vi "Main.vi"() -> ()   [LabVIEW 2017]
doc: "The myRIO Project template acquires acceleration data from the onboard accelerometer and displays the changes of acceleration values in a waveform chart."
uses:
  <vilib>/myRIO/Common/Instrument Driver Framework/myRIO v1.0/IRQ/typedefs/DI IRQ Type.ctl
  <vilib>/Platform/TimedLoop/XDataNode/timing_clust.ctl
  <vilib>/Platform/TimedLoop/XDataNode/nitl_modes.ctl
  <vilib>/Platform/TimedLoop/XDataNode/wakeup.ctl
  <vilib>/myRIO/Common/Instrument Driver Framework/myRIO v1.0/Encoder/typedefs/Encoder Signal Mode.ctl
  <vilib>/myRIO/Instrument Drivers/Onboard IO/Encoder/typedefs/Encoder Reference.ctl
  <vilib>/myRIO/Common/Instrument Driver Framework/Utilities/typedefs/myRIO Generic Hardware Reference.ctl
  <vilib>/myRIO/Common/Instrument Driver Framework/Utilities/typedefs/Hardware Version Enum.ctl
  <vilib>/myRIO/Common/Instrument Driver Framework/Utilities/typedefs/myRIO v1.0 Reference.ctl
  <vilib>/myRIO/Common/Instrument Driver Framework/Utilities/typedefs/Generic FPGA Reference.ctl
  <vilib>/myRIO/Common/Instrument Driver Framework/myRIO v1.0/Encoder/typedefs/Encoder Channels Enum.ctl
  <vilib>/myRIO/Common/Instrument Driver Framework/myRIO v1.0/Encoder/typedefs/Encoder Configuration v1.0.ctl
  <vilib>/userdefined/High Color/nirio_resource_hc.ctl
  <vilib>/myRIO/Instrument Drivers/Onboard IO/DIO/typedefs/DIO Reference.ctl
  <vilib>/myRIO/Common/Instrument Driver Framework/myRIO v1.0/DIO/typedefs/DIO Channels List.ctl
  <vilib>/myRIO/Common/Instrument Driver Framework/myRIO v1.0/DIO/typedefs/DIO Channels Enum.ctl
  <vilib>/myRIO/Instrument Drivers/Onboard Devices/Accelerometer/typedefs/Accelerometer Reference.ctl
  <vilib>/myRIO/Common/Instrument Driver Framework/myRIO v1.0/Accelerometer/typedefs/Accelerometer Channels List.ctl
  <vilib>/myRIO/Common/Instrument Driver Framework/myRIO v1.0/Accelerometer/typedefs/Accelerometer Channels Enum.ctl
  <vilib>/myRIO/Common/Instrument Driver Framework/Utilities/vis/Is FPGA Ref Available.vi
  <vilib>/myRIO/Common/Instrument Driver Framework/myRIO v1.0/Encoder/vis/myRIO v1.1 Open Encoder.vi
  <vilib>/myRIO/Instrument Drivers/Onboard IO/Encoder/vis/Read.vi
  <vilib>/myRIO/Common/Instrument Driver Framework/myRIO v1.0/Accelerometer/vis/myRIO v1.1 Open Accelerometer.vi
  <vilib>/myRIO/Instrument Drivers/Onboard Devices/Accelerometer/vis/Read.vi
  <vilib>/myRIO/Common/Instrument Driver Framework/myRIO v1.0/DIO/vis/myRIO v1.1 Open DIO.vi
  <vilib>/myRIO/Instrument Drivers/Onboard IO/DIO/vis/Read.vi
  <vilib>/myRIO/Instrument Drivers/Onboard IO/DIO/vis/Write.vi
  <vilib>/myRIO/Common/Instrument Driver Framework/Utilities/vis/Validate Channels.vi
  <vilib>/myRIO/Common/Instrument Driver Framework/myRIO v1.0/Encoder/vis/myRIO v1.0 Reserve Encoder.vi
  <vilib>/myRIO/Common/Instrument Driver Framework/myRIO v1.0/UART/vis/myRIO v1.0 Close UART.vi
  <vilib>/myRIO/Common/Instrument Driver Framework/myRIO v1.0/Accelerometer/vis/myRIO v1.0 Reserve Accelerometer.vi
  <vilib>/myRIO/Common/Instrument Driver Framework/myRIO v1.0/DIO/vis/myRIO v1.0 Reserve DIO.vi
  <vilib>/myRIO/Common/Instrument Driver Framework/myRIO v1.0/Encoder/vis/myRIO v1.0 Build MUX Configuration Encoder.vi
  <vilib>/myRIO/Common/Instrument Driver Framework/myRIO v1.0/Resource Manager/vis/myRIO v1.0 Reserve Channel List.vi
  <vilib>/myRIO/Common/Instrument Driver Framework/myRIO v1.0/Accelerometer/vis/myRIO v1.0 Build MUX Configuration Accelerometer.vi
  <vilib>/myRIO/Common/Instrument Driver Framework/myRIO v1.0/DIO/vis/myRIO v1.0 Build MUX Configuration DIO.vi
  <vilib>/myRIO/Common/Instrument Driver Framework/myRIO v1.0/Resource Manager/vis/myRIO v1.0 Create Configuration List.vi
  <vilib>/myRIO/Common/Instrument Driver Framework/myRIO v1.0/Resource Manager/vis/myRIO v1.0 Reserve Channel.vi
  <vilib>/myRIO/Common/Instrument Driver Framework/myRIO v1.0/Resource Manager/vis/myRIO v1.0 Unreserve Channel.vi
  <vilib>/myRIO/Common/Instrument Driver Framework/myRIO v1.0/Resource Manager/vis/myRIO v1.0 Build Mutex Name.vi
  global.vi
  <vilib>/Utility/VariantDataType/GetNumericInfo.vi
  <vilib>/Utility/error.llb/Error Cluster From Error Code.vi
  <vilib>/myRIO/Common/Instrument Driver Framework/myRIO v1.0/myRIO v1.1 Open.vi
  <vilib>/myRIO/Common/Instrument Driver Framework/Utilities/vis/IO Manager.vi
  <vilib>/myRIO/Common/Instrument Driver Framework/Utilities/vis/Configuration Manager.vi
  <vilib>/myRIO/Common/Instrument Driver Framework/myRIO v1.0/Resource Manager/vis/myRIO v1.0 Configure IO.vi
  <vilib>/myRIO/Common/Instrument Driver Framework/myRIO v1.0/myRIO v1.0 Close.vi
  <vilib>/myRIO/Common/Instrument Driver Framework/myRIO v1.0/Encoder/vis/myRIO v1.0 Configure Encoder.vi
  <vilib>/myRIO/Common/Instrument Driver Framework/myRIO v1.0/Encoder/vis/myRIO v1.0 Read Encoder.vi
  State2016.vi
  <vilib>/addons/control/pid/pid.llb/PID (DBL).vi
  <vilib>/myRIO/Common/Instrument Driver Framework/Utilities/vis/FPGA Ref Manager.vi
  <vilib>/myRIO/Common/Instrument Driver Framework/myRIO v1.0/myRIO v1.0 Reset FPGA.vi
  <vilib>/myRIO/Common/Instrument Driver Framework/myRIO v1.0/IRQ/vis/myRIO v1.0 IRQ Info FGV.vi
  <vilib>/myRIO/Common/Instrument Driver Framework/myRIO v1.0/IRQ/vis/myRIO v1.0 Timer IRQ Info FGV.vi
  <vilib>/myRIO/Common/Instrument Driver Framework/myRIO v1.0/IRQ/vis/myRIO v1.0 ISR Agent.vi
  motion_command.vi
  <vilib>/myRIO/Common/Instrument Driver Framework/myRIO v1.0/DIO/vis/myRIO v1.0 Write DIO.vi
  <vilib>/myRIO/Common/Instrument Driver Framework/myRIO v1.0/DIO/vis/myRIO v1.0 Read DIO.vi
  <vilib>/myRIO/Common/Instrument Driver Framework/myRIO v1.0/Accelerometer/vis/myRIO v1.0 Get Scaling Constant Accelerometer.vi
  <vilib>/myRIO/Common/Instrument Driver Framework/myRIO v1.0/Accelerometer/vis/myRIO v1.0 Read Accelerometer.vi
  <vilib>/myRIO/Common/Instrument Driver Framework/myRIO v1.0/IRQ/vis/myRIO v1.1 Register DI IRQ.vi
  <vilib>/Platform/TimedLoop/XDataNode/XDataNode.xnode
  <vilib>/myRIO/Express VI/Onboard IO/Encoder/Encoder Express VI.xnode
  <vilib>/myRIO/Instrument Drivers/Onboard IO/Encoder/vis/myRIO Encoder Open.xnode
  <vilib>/myRIO/Common/Instrument Driver Framework/myRIO v1.0/Encoder/typedefs/Encoder Count Direction Enum.ctl
  <vilib>/myRIO/Express VI/Onboard Devices/LED/LED Express VI.xnode
  <vilib>/myRIO/Instrument Drivers/Onboard IO/DIO/vis/myRIO DIO Open.xnode
  <vilib>/myRIO/Express VI/Onboard IO/DI/DI Express VI.xnode
  <vilib>/myRIO/Express VI/Onboard Devices/Accelerometer/Accelerometer Express VI.xnode
  <vilib>/myRIO/Instrument Drivers/Onboard Devices/Accelerometer/vis/myRIO Accelerometer Open.xnode
  <vilib>/myRIO/Instrument Drivers/IRQ/IO IRQ/vis/myRIO Register DI IRQ.xnode
  <vilib>/myRIO/Common/Instrument Driver Framework/myRIO v1.0/IRQ/typedefs/Callback VI Ref.ctl
  <vilib>/myRIO/Instrument Drivers/Utilities/Utilities.lvlib
  <vilib>/Platform/TimedLoop/XDataNode/XDNodeRunTimeDep.lvlib
  <vilib>/myRIO/Instrument Drivers/Onboard IO/Encoder/Encoder.lvlib
  <vilib>/addons/control/pid/NI_PID_pid.lvlib
  <vilib>/myRIO/Instrument Drivers/Onboard IO/DIO/DIO.lvlib
  <vilib>/myRIO/Instrument Drivers/Onboard Devices/Accelerometer/Accelerometer.lvlib
panel:
  in  "T/S":bool
  in  "Speed":dbl(slide) scale=0.0..1.0
  in  "Torque":dbl(slide) scale=0.0..500.0
  out "Motion\nCommand":bool
  out "S/T Control":bool
  in  "Speed scale":dbl=1.0 format="%#_13g"
  in  "Stop":bool
  out "error out 2":errorcluster
  in  "PID gains 2":T1={"proportional gain (Kc)"=150.0, "integral time (Ti, min)"=0.0005, "derivative time (Td, min)"=1e-06} caption="PID 게인" {"derivative time (Td, min)" format="%.6f"; "integral time (Ti, min)" format="%.4f"; "proportional gain (Kc)" format="%.3f"}
  out "웨이브폼 차트 2":cluster{"Speed":dbl, dbl, dbl}(graph)={"Speed"=0.003129890453834161, -6.70631856770996, 0.00312989045383416}
  out "m/s 2":dbl(knob)=6.70631856770996 scale=0.0..2.0
  out "RPS 2":dbl(knob)=14.23125 scale=0.0..5.0
  out "km/h 2":dbl(knob)=24.14274684375586 scale=0.0..10.0
  out "RPM 2":dbl(knob)=853.875 scale=0.25..250.0
  out "output 2":dbl=500.0
  out "CW 2":bool
  in  "ip 2":i32=77
  out "RC Control":bool
  out "CW":bool
  out "output":dbl=-44.009136764238946
  out "RPM":dbl(knob)=0.75 scale=0.25..250.0
  out "km/h":dbl(knob)=0.021205750411731103 scale=0.0..10.0
  out "RPS":dbl(knob)=0.0125 scale=0.0..5.0
  out "m/s":dbl(knob)=0.005890486225480862 scale=0.0..2.0
  out "웨이브폼 차트":cluster{"Speed":dbl, dbl, dbl}(graph)={"Speed"=0.003129890453834161, 0.005890486225480862, 0.00312989045383416}
  in  "PID gains":T1={"proportional gain (Kc)"=150.0, "integral time (Ti, min)"=0.0005, "derivative time (Td, min)"=1e-06} caption="PID 게인" {"derivative time (Td, min)" format="%.6f"; "integral time (Ti, min)" format="%.4f"; "proportional gain (Kc)" format="%.3f"}
  in  "ip":i32=76
  out "error out":errorcluster
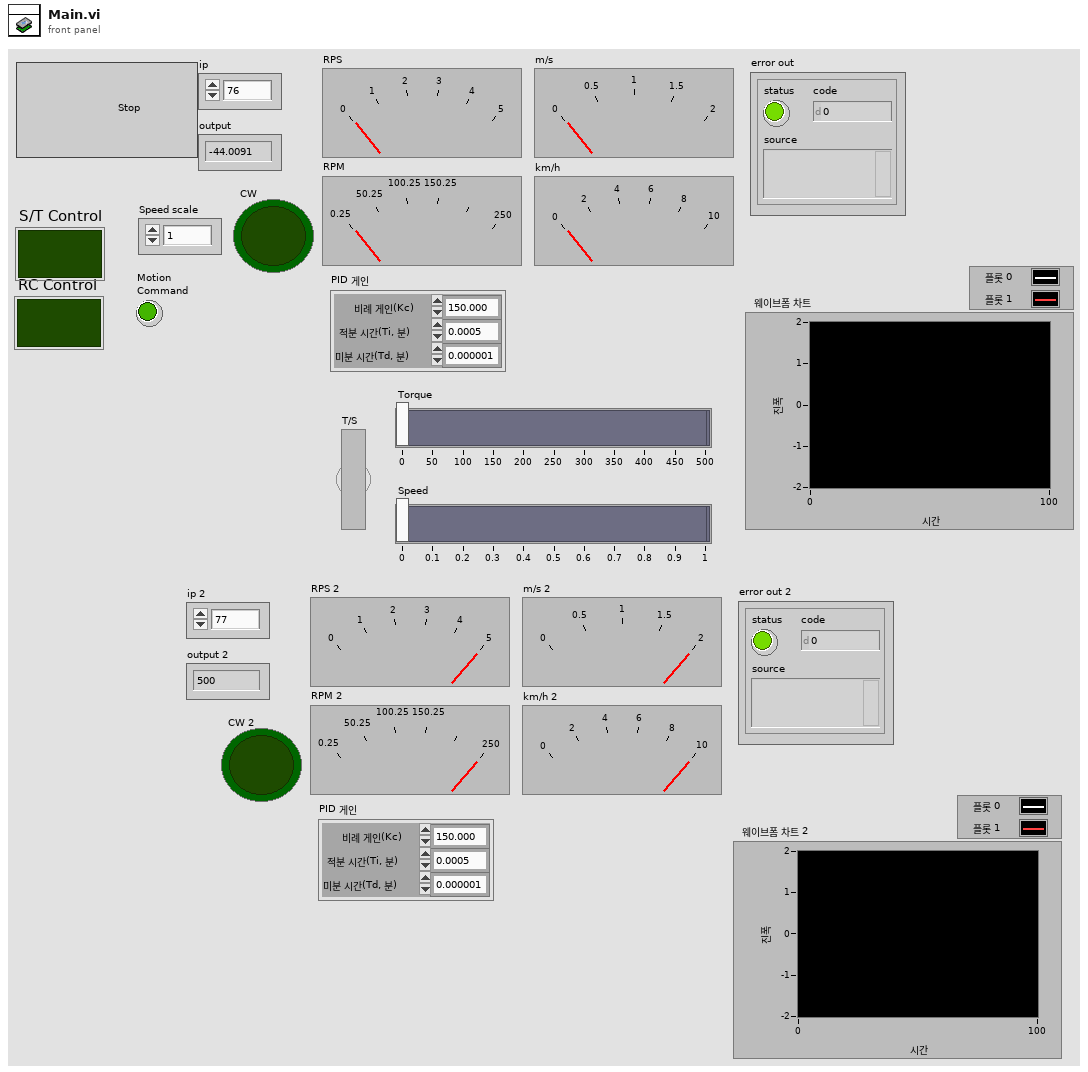
[diagram p1: front panel]
types:
  T1 = cluster{"proportional gain (Kc)":dbl, "integral time (Ti, min)":dbl, "derivative time (Td, min)":dbl}
  T2 = typedef "DI IRQ Type.ctl" = enum16{"Digital falling edge", "Digital rising edge", "Digital edge"}
  T3 = typedef "XDNodeRunTimeDep.lvlib/timing_clust.ctl" = cluster{"Expected End [f-1]":u64, "Actual End [f-1]":u64, "Finished Late? [f-1]":bool, "Expected End [i-1]":u64, "Actual End [i-1]":u64, "Finished Late? [i-1]":bool, "Expected Start [i]":u64, "Actual Start [i]":u64, "Expected Start [f]":u64, "Actual Start [f]":u64, "Source Name":string, "Structure Name":string, "Period":i64, "Deadline":i64, "Offset":i64, "Start":i64, "Priority":i32, "Timeout":i32, "Mode":T4, "Wakeup Reason":T5, "Error":errorcluster, "Source Type":string, "Secondary Source Type":string, "Global End Time":u64, "Global Start Time":u64, "Frame Duration":u64, "Iteration Duration":u64, "Assigned CPU":i32, "I/O Scan Engine Mode":u32}
  T4 = typedef "XDNodeRunTimeDep.lvlib/nitl_modes.ctl" = enum32{"No Change", "Process missed periods, maintain original phase", "Discard missed periods, maintain original phase", "Process missed periods, ignore original phase", "Discard missed periods, ignore original phase"}
  T5 = typedef "XDNodeRunTimeDep.lvlib/wakeup.ctl" = enum32{"Normal", "Aborted", "Asynchronous wakeup", "Timing source error", "Timed loop error", "Timeout"}
  T6 = typedef "Encoder.lvlib/Encoder Reference.ctl" = cluster{"myRIO Reference":T7, "Encoder Channels Enum":T11}
  T7 = typedef "myRIO Generic Hardware Reference.ctl" = cluster{"myRIO Model":T8, "myRIO Hardware Reference":T9}
  T8 = typedef "Hardware Version Enum.ctl" = enum16{"Unknown", "myRIO-1900", "myRIO-1950", "roboRIO", "NI ELVIS RIO CM"}
  T9 = typedef "myRIO v1.0 Reference.ctl" = cluster{"Generic FPGA Reference":T10, "Allow multiple opens":bool}
  T10 = typedef "Generic FPGA Reference.ctl" = refnum<k20>
  T11 = typedef "Encoder Channels Enum.ctl" = enum16{"Not Connected", "C/ENC0", "C/ENC1", "A/ENC", "B/ENC", "DIO/ENC0", "DIO/ENC1", "DIO/ENC2", "DIO/ENC3", "DIO/ENC4"}
  T12 = typedef "Encoder Signal Mode.ctl" = enum16{"Quadrature phase signal", "Step and direction signal"}
  T13 = typedef "nirio_resource_hc.ctl" = tag
  T14 = typedef "Accelerometer.lvlib/Accelerometer Reference.ctl" = cluster{"myRIO Reference":T7, "Accelerometer Channels List":T15, "LSB Weight":dbl}
  T15 = typedef "Accelerometer Channels List.ctl" = T16[]
  T16 = typedef "Accelerometer Channels Enum.ctl" = enum16{"Not Connected", "X-Axis", "Y-Axis", "Z-Axis"}
  T17 = typedef "DIO.lvlib/DIO Reference.ctl" = cluster{"myRIO Reference":T7, "DIO Channels List":T18}
  T18 = typedef "DIO Channels List.ctl" = T19[]
  T19 = typedef "DIO Channels Enum.ctl" = enum16{"Not Connected", "C/DIO0", "C/DIO1", "C/DIO2", "C/DIO3", "C/DIO4", "C/DIO5", "C/DIO6", "C/DIO7", "A/DIO0", "A/DIO1", "A/DIO2", "A/DIO3", "A/DIO4", "A/DIO5", "A/DIO6", "A/DIO7", "A/DIO8", "A/DIO9", "A/DIO10", "A/DIO11", "A/DIO12", "A/DIO13", "A/DIO14", "A/DIO15", "B/DIO0", "B/DIO1", "B/DIO2", "B/DIO3", "B/DIO4", "B/DIO5", "B/DIO6", "B/DIO7", "B/DIO8", "B/DIO9", "B/DIO10", "B/DIO11", "B/DIO12", "B/DIO13", "B/DIO14", "B/DIO15", "LED0", "LED1", "LED2", "LED3", "Button0", "DIO/DIO0", "DIO/DIO1", "DIO/DIO2", "DIO/DIO3", "DIO/DIO4", "DIO/DIO5", "DIO/DIO6", "DIO/DIO7", "DIO/DIO8", "DIO/DIO9", "SPI/CS0", "SPI/CS1", "SPI/CS2", "SPI/CS3", "LED RADIO (Green)", "LED RADIO (Red)", "LED COMM (Green)", "LED COMM (Red)", "LED MODE (Green)", "LED MODE (Red)"}
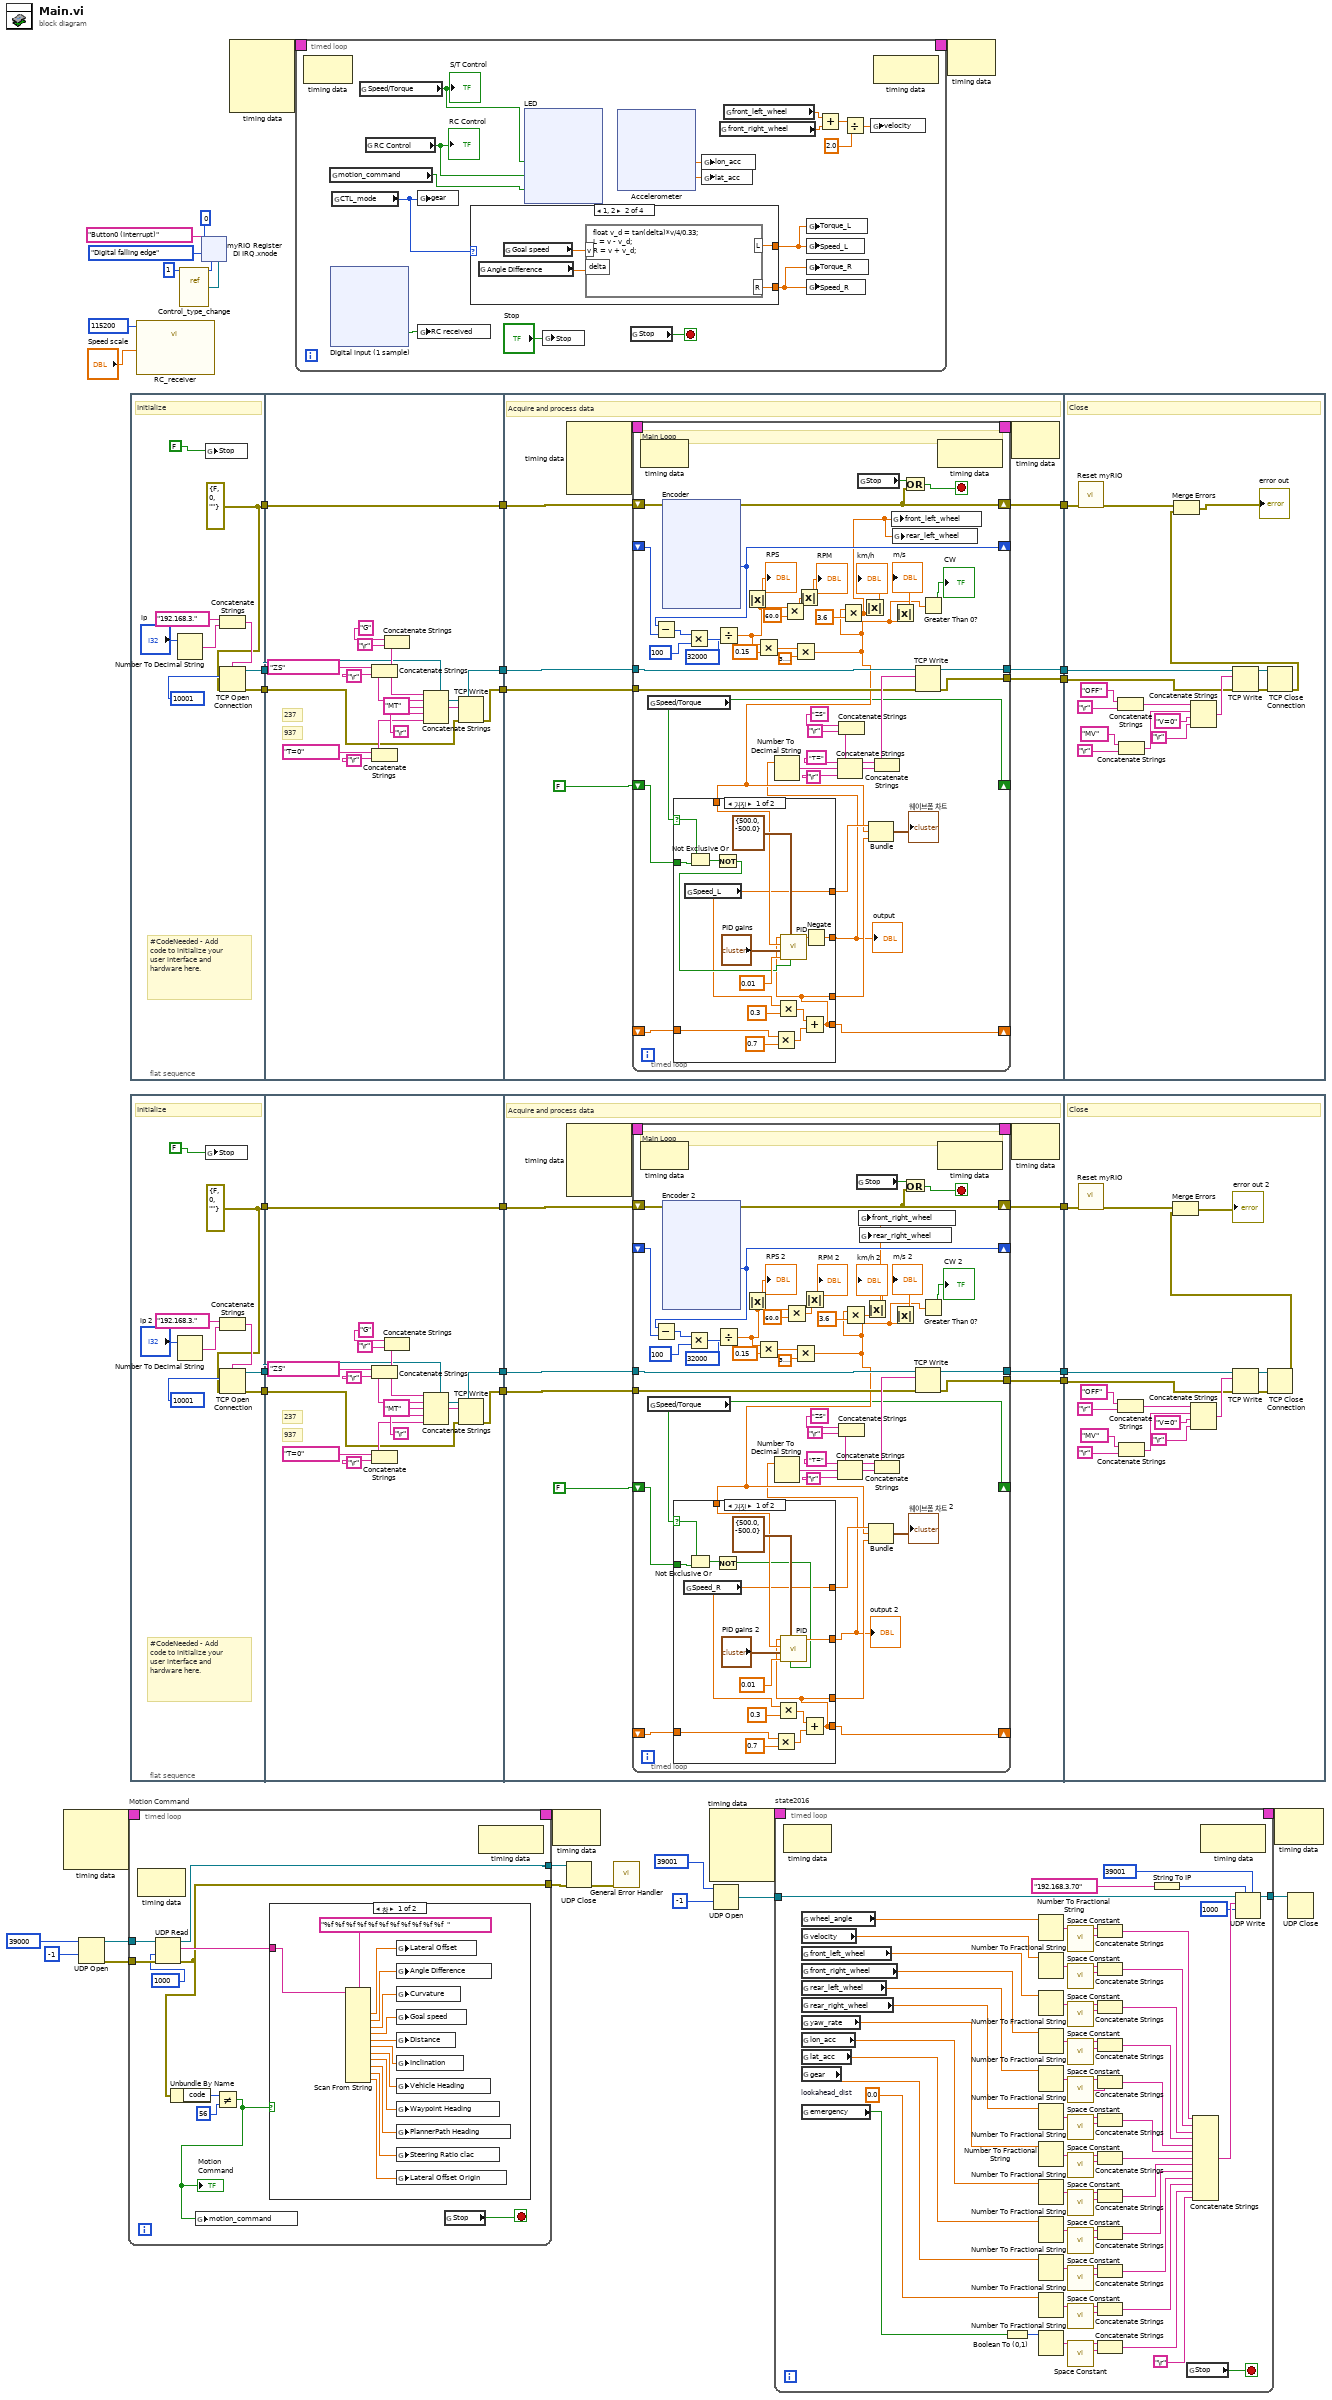
[diagram p0: block diagram]
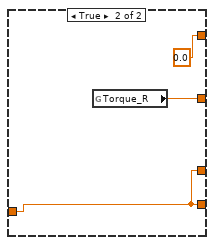
[diagram p3: hidden frame]
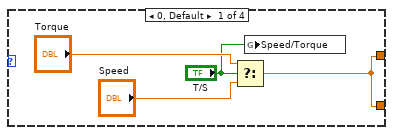
[diagram p4: hidden frame]
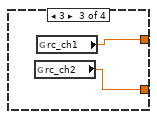
[diagram p5: hidden frame]
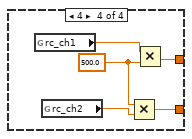
[diagram p6: hidden frame]
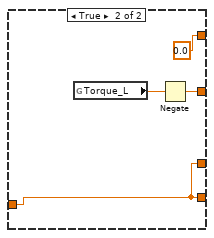
[diagram p7: hidden frame]
diagram:
  n1 = node-c288() -> (w17:T3)  [unwired: 3 in]
  n2 = UDP Open(9:-1 ("타임아웃 ms (25000)"), 11:u16 39000 ("포트")) -> (port=w15:refnum<k16>, 0:w11:errorcluster)  [unwired: 3 in, 1 out]
  n3 = timed-loop "Motion Command" {
    tunnel: w15 -> [w52]
    tunnel: [w46] -> w14
    timing: w17 -> [_]
    timing-out: [_] -> w16
    tunnel: w11 -> [w50]
    tunnel: [w47] -> w10
    stop <- w45 stop-if-true
    n4 = node-c288() -> ()  [unwired: 1 in, 1 out]
    n5 = UDP Read(connection ID=w52, timeout ms (25000)=1000 ("타임아웃 ms (25000)"), 8:w50) -> (data out=w51:string, error out=w47:errorcluster, 3:w46:refnum<k16>)  [unwired: 1 in, 2 out]
    n6 = Unbundle By Name(w47) -> ("code"=w49:i32)
    n7 = Not Equal?(x=w49, y=56) -> (x != y?=w44:bool)
    "Motion\nCommand" <- w44
    n8 = global write "global.vi" "motion_command"(w44) -> ()
    n9 = case shown="참" w44 {
      tunnel: w51 -> [w64 _]
      frame True {
        n10 = Scan From String(format string="%f %f %f %f %f %f %f %f %f %f %f  " ("포맷 문자열"), input string=w64) -> (output 1=w58:dbl, output 2=w60:dbl, output 3=w59:dbl, output 4=w62:dbl, output 5=w63:dbl, output 6=w61:dbl, output 7=w55:dbl, output 8=w54:dbl, output 9=w53:dbl, output 10=w56:dbl, output 11=w57:dbl)  [unwired: 13 in, 3 out]
        n11 = global write "motion_command.vi" "Lateral Offset"(w58) -> ()
        n12 = global write "motion_command.vi" "Angle Difference"(w60) -> ()
        n13 = global write "motion_command.vi" "Curvature"(w59) -> ()
        n14 = global write "motion_command.vi" "Goal speed"(w62) -> ()
        n15 = global write "motion_command.vi" "Distance"(w63) -> ()
        n16 = global write "motion_command.vi" "Inclination"(w61) -> ()
        n17 = global write "motion_command.vi" "Vehicle Heading"(w55) -> ()
        n18 = global write "motion_command.vi" "Waypoint Heading"(w54) -> ()
        n19 = global write "motion_command.vi" "PlannerPath Heading"(w53) -> ()
        n20 = global write "motion_command.vi" "Steering Ratio clac"(w56) -> ()
        n21 = global write "motion_command.vi" "Lateral Offset Origin"(w57) -> ()
      }
      frame False {
      }
    }
    n22 = global read "global.vi" "Stop"() -> (w45:bool)
    n23 = node-c288() -> ()  [unwired: 1 in, 1 out]
  }
  n24 = flat-sequence {
    tunnel: [w69] -> w41
    tunnel: [w75] -> w39
    tunnel: [w70] -> w36
    tunnel: w41 -> [w93]
    tunnel: [w93] -> w40
    tunnel: w39 -> [w80]
    tunnel: [w79] -> w38
    tunnel: w36 -> [w77]
    tunnel: [w78] -> w35
    tunnel: w40 -> [w102]
    tunnel: [w101] -> w42
    tunnel: w38 -> [w100]
    tunnel: [w97] -> w37
    tunnel: w35 -> [w96]
    tunnel: [w95] -> w34
    tunnel: w42 -> [w234]
    tunnel: w37 -> [w223]
    tunnel: w34 -> [w222]
    frame #0 {
      w69 = errorcluster {"status"=FALSE, "code"=0, "source"=""} ("error in (no error)")
      # "#CodeNeeded - Add code to initialize your user interface and hardware here."
      # "Initialize"
      n25 = Number To Decimal String(number="ip") -> (decimal integer string=w72:string)  [unwired: 1 in]
      n26 = global write "global.vi" "Stop"(FALSE ("status")) -> ()
      n27 = Concatenate Strings("192.168.3." ("주소"), w72) -> (w73:string)
      n28 = TCP Open Connection(address=w73, remote port or service name=u16 10001 ("원격 포트 또는 서비스 이름"), error in (no error)=w69) -> (connection ID=w75:refnum<k5>, error out=w70:errorcluster)  [unwired: 2 in]
    }
    frame #1 {
      # "937"
      # "237"
      n29 = Concatenate Strings("ZS" ("데이터 입력"), "\r") -> (w88:string)
      n30 = Concatenate Strings("T=0" ("데이터 입력"), "\r") -> (w89:string)
      n31 = Concatenate Strings("G" ("문자열"), "\r") -> (w81:string)
      n32 = Concatenate Strings(w81, w88, "MT" ("데이터 입력"), "\r", w89) -> (w84:string)
      n33 = TCP Write(connection ID=w80, data in=w84, error in (no error)=w77) -> (connection ID out=w79:refnum<k5>, error out=w78:errorcluster)  [unwired: 1 in, 1 out]
    }
    frame #2 {
      # "Acquire and process data"
      n34 = node-c288() -> (w99:T3)  [unwired: 4 in]
      n35 = timed-loop {
        shift-right: [w108] -> w101
        shift-left: w102 -> [w133]
        tunnel: w100 -> [w138]
        timing: w99 -> [_]
        timing-out: [_] -> w98
        tunnel: [w137] -> w97
        tunnel: w96 -> [w136]
        tunnel: [w134] -> w95
        shift-right: [w127] -> _
        shift-left: _ -> [w132]
        shift-right: [w107] -> _
        shift-left: FALSE ("Speed/Torque") -> [w124]
        shift-right: [w117] -> _
        shift-left: _ -> [w118]
        stop <- w135 stop-if-true
        # "Main Loop"
        n36 = node-c288() -> ()  [unwired: 1 in, 1 out]
        n37 = global read "global.vi" "Speed/Torque"() -> (w107:bool)
        n38 = xnode "Encoder"("error in (no error)"=w133) -> ("Counter Value"=w127:i32, "error out"=w108:errorcluster)  [unwired: 1 in, 2 out]
        n39 = Subtract(x=w127, y=w132) -> (x-y=w131:i32)
        n40 = Multiply(x=w131, y=100) -> (x*y=w129:i32)
        n41 = Divide(x=w129, y=32000) -> (x/y=w105:dbl)
        n42 = Absolute Value(x=w105) -> (abs(x)=→"RPS":dbl)
        n43 = Multiply(x=w105, y=0.15) -> (x*y=w122:dbl)
        n44 = Multiply(x=w105, y=60.0) -> (x*y=w104:dbl)
        n45 = Multiply(x=w122, y=3.141592653589793) -> (x*y=w111:dbl)
        n46 = case shown="거짓" w107 {
          selector: w107 -> [w157 _]
          tunnel: [w148 w165] -> w106
          tunnel: w111 -> [w160 _]
          tunnel: [w147 0.0 ("Speed")] -> w125
          tunnel: w124 -> [w156 _]
          tunnel: w118 -> [w151 w166]
          tunnel: [w150 w166] -> w117
          tunnel: [w150 w166] -> w116
          frame False {
            n47 = global read "global.vi" "Speed_L"() -> (w147:dbl)
            n48 = Not Exclusive Or(1:w156, 2:w157) -> (0:w159:bool)
            n49 = Not(x=w159) -> (.not. x?=w158:bool)
            n50 = Multiply(x=w151, y=0.7) -> (x*y=w155:dbl)
            n51 = Multiply(x=w147, y=0.3) -> (x*y=w154:dbl)
            n52 = Add(x=w154, y=w155) -> (x+y=w150:dbl)
            n53 = call-poly <vilib>:"PID.vi"("reinitialize? (F)"=w158, "output range"=cluster{"output high":dbl, "output low":dbl} {"output high"=500.0, "output low"=-500.0}, "dt (s)"=0.01, "PID gains"="PID gains", "process variable"=w160, "setpoint"=w150) -> ("output"=w149:dbl)  [unwired: 4 in, 1 out]
            n54 = Negate(x=w149) -> (-x=w148:dbl)
          }
          frame True {
            n55 = global read "global.vi" "Torque_L"() -> (w164:dbl)
            n56 = Negate(x=w164) -> (-x=w165:dbl)
          }
        }
        "output" <- w106
        n57 = Number To Decimal String(number=w106) -> (decimal integer string=w140:string)  [unwired: 1 in]
        n58 = Absolute Value(x=w104) -> (abs(x)=→"RPM":dbl)
        n59 = Concatenate Strings("T=", w140, "\r") -> (w144:string)
        n60 = Concatenate Strings("ZS", "\r") -> (w141:string)
        n61 = Multiply(x=w111, y=3.6) -> (x*y=w103:dbl)
        n62 = global read "global.vi" "Stop"() -> (w109:bool)
        n63 = Absolute Value(x=w103) -> (abs(x)=→"km/h":dbl)
        n64 = Bundle("Speed"=w125, w111, w116) -> (→"웨이브폼 차트":cluster{"Speed":dbl, dbl, dbl})  [unwired: 1 in]
        n65 = Concatenate Strings(w141, w144) -> (w139:string)
        n66 = global write "State2016.vi" "front_left_wheel"(w103) -> ()
        n67 = global write "State2016.vi" "rear_left_wheel"(w103) -> ()
        n68 = Absolute Value(x=w111) -> (abs(x)=→"m/s":dbl)
        n69 = Or(x=w109, y=w108) -> (x .or. y?=w135:bool)
        n70 = TCP Write(connection ID=w138, data in=w139, error in (no error)=w136) -> (connection ID out=w137:refnum<k5>, error out=w134:errorcluster)  [unwired: 1 in, 1 out]
        n71 = Greater Than 0?(x=w111) -> (x > 0?=→"CW":bool)
        n72 = node-c288() -> ()  [unwired: 1 in, 1 out]
      }
      n73 = node-c288(w98) -> ()  [unwired: 1 out]
    }
    frame #3 {
      # "Close"
      n74 = call <vilib>:"Reset myRIO.vi"("error in (no error)"=w234) -> ("error out"=w219:errorcluster)  [unwired: 10 in]
      n75 = Concatenate Strings("OFF" ("데이터 입력"), "\r") -> (w228:string)
      n76 = Concatenate Strings("MV" ("데이터 입력"), "\r") -> (w227:string)
      n77 = Concatenate Strings(w228, w227, "V=0" ("데이터 입력"), "\r") -> (w224:string)
      n78 = TCP Write(connection ID=w223, data in=w224, error in (no error)=w222) -> (connection ID out=w233:refnum<k5>, error out=w221:errorcluster)  [unwired: 1 in, 1 out]
      n79 = TCP Close Connection(connection ID=w233, error in (no error)=w221) -> (error out=w218:errorcluster)  [unwired: 1 in, 1 out]
      n80 = Merge Errors(w219, w218) -> (→"error out":errorcluster)
    }
  }
  n81 = flat-sequence {
    tunnel: [w236] -> w26
    tunnel: [w242] -> w25
    tunnel: [w237] -> w24
    tunnel: w26 -> [w260]
    tunnel: [w260] -> w23
    tunnel: w25 -> [w247]
    tunnel: [w246] -> w22
    tunnel: w24 -> [w244]
    tunnel: [w245] -> w21
    tunnel: w23 -> [w269]
    tunnel: [w268] -> w20
    tunnel: w22 -> [w267]
    tunnel: [w264] -> w19
    tunnel: w21 -> [w263]
    tunnel: [w262] -> w18
    tunnel: w20 -> [w399]
    tunnel: w19 -> [w388]
    tunnel: w18 -> [w387]
    frame #0 {
      w236 = errorcluster {"status"=FALSE, "code"=0, "source"=""} ("error in (no error)")
      # "#CodeNeeded - Add code to initialize your user interface and hardware here."
      # "Initialize"
      n82 = Number To Decimal String(number="ip 2") -> (decimal integer string=w239:string)  [unwired: 1 in]
      n83 = global write "global.vi" "Stop"(FALSE ("status")) -> ()
      n84 = Concatenate Strings("192.168.3." ("주소"), w239) -> (w240:string)
      n85 = TCP Open Connection(address=w240, remote port or service name=u16 10001 ("원격 포트 또는 서비스 이름"), error in (no error)=w236) -> (connection ID=w242:refnum<k5>, error out=w237:errorcluster)  [unwired: 2 in]
    }
    frame #1 {
      # "937"
      # "237"
      n86 = Concatenate Strings("ZS" ("데이터 입력"), "\r") -> (w255:string)
      n87 = Concatenate Strings("T=0" ("데이터 입력"), "\r") -> (w256:string)
      n88 = Concatenate Strings("G" ("문자열"), "\r") -> (w248:string)
      n89 = Concatenate Strings(w248, w255, "MT" ("데이터 입력"), "\r", w256) -> (w251:string)
      n90 = TCP Write(connection ID=w247, data in=w251, error in (no error)=w244) -> (connection ID out=w246:refnum<k5>, error out=w245:errorcluster)  [unwired: 1 in, 1 out]
    }
    frame #2 {
      # "Acquire and process data"
      n91 = node-c288() -> (w266:T3)  [unwired: 4 in]
      n92 = timed-loop {
        shift-right: [w274] -> w268
        shift-left: w269 -> [w300]
        tunnel: w267 -> [w305]
        timing: w266 -> [_]
        timing-out: [_] -> w265
        tunnel: [w304] -> w264
        tunnel: w263 -> [w303]
        tunnel: [w301] -> w262
        shift-right: [w294] -> _
        shift-left: _ -> [w299]
        shift-right: [w273] -> _
        shift-left: FALSE ("Speed/Torque") -> [w291]
        shift-right: [w283] -> _
        shift-left: _ -> [w284]
        stop <- w302 stop-if-true
        # "Main Loop"
        n93 = node-c288() -> ()  [unwired: 1 in, 1 out]
        n94 = global read "global.vi" "Speed/Torque"() -> (w273:bool)
        n95 = xnode "Encoder 2"("error in (no error)"=w300) -> ("Counter Value"=w294:i32, "error out"=w274:errorcluster)  [unwired: 1 in, 2 out]
        n96 = Subtract(x=w294, y=w299) -> (x-y=w298:i32)
        n97 = Multiply(x=w298, y=100) -> (x*y=w296:i32)
        n98 = Divide(x=w296, y=32000) -> (x/y=w288:dbl)
        n99 = Absolute Value(x=w288) -> (abs(x)=→"RPS 2":dbl)
        n100 = Multiply(x=w288, y=0.15) -> (x*y=w289:dbl)
        n101 = Multiply(x=w288, y=60.0) -> (x*y=w271:dbl)
        n102 = Multiply(x=w289, y=3.141592653589793) -> (x*y=w277:dbl)
        n103 = case shown="거짓" w273 {
          selector: w273 -> [w322 _]
          tunnel: [w326 w330] -> w272
          tunnel: w277 -> [w325 _]
          tunnel: [w314 0.0 ("Speed")] -> w292
          tunnel: w291 -> [w321 _]
          tunnel: w284 -> [w316 w331]
          tunnel: [w315 w331] -> w283
          tunnel: [w315 w331] -> w282
          frame False {
            n104 = global read "global.vi" "Speed_R"() -> (w314:dbl)
            n105 = Not Exclusive Or(1:w321, 2:w322) -> (0:w324:bool)
            n106 = Not(x=w324) -> (.not. x?=w323:bool)
            n107 = Multiply(x=w316, y=0.7) -> (x*y=w320:dbl)
            n108 = Multiply(x=w314, y=0.3) -> (x*y=w319:dbl)
            n109 = Add(x=w319, y=w320) -> (x+y=w315:dbl)
            n110 = call-poly <vilib>:"PID.vi"("reinitialize? (F)"=w323, "output range"=cluster{"output high":dbl, "output low":dbl} {"output high"=500.0, "output low"=-500.0}, "dt (s)"=0.01, "PID gains"="PID gains 2", "process variable"=w325, "setpoint"=w315) -> ("output"=w326:dbl)  [unwired: 4 in, 1 out]
          }
          frame True {
            n111 = global read "global.vi" "Torque_R"() -> (w330:dbl)
          }
        }
        "output 2" <- w272
        n112 = Number To Decimal String(number=w272) -> (decimal integer string=w307:string)  [unwired: 1 in]
        n113 = Absolute Value(x=w271) -> (abs(x)=→"RPM 2":dbl)
        n114 = Concatenate Strings("T=", w307, "\r") -> (w311:string)
        n115 = Concatenate Strings("ZS", "\r") -> (w308:string)
        n116 = Multiply(x=w277, y=3.6) -> (x*y=w270:dbl)
        n117 = global read "global.vi" "Stop"() -> (w275:bool)
        n118 = global write "State2016.vi" "front_right_wheel"(w270) -> ()
        n119 = global write "State2016.vi" "rear_right_wheel"(w270) -> ()
        n120 = Absolute Value(x=w270) -> (abs(x)=→"km/h 2":dbl)
        n121 = Bundle("Speed"=w292, w277, w282) -> (→"웨이브폼 차트 2":cluster{"Speed":dbl, dbl, dbl})  [unwired: 1 in]
        n122 = Concatenate Strings(w308, w311) -> (w306:string)
        n123 = Absolute Value(x=w277) -> (abs(x)=→"m/s 2":dbl)
        n124 = Or(x=w275, y=w274) -> (x .or. y?=w302:bool)
        n125 = TCP Write(connection ID=w305, data in=w306, error in (no error)=w303) -> (connection ID out=w304:refnum<k5>, error out=w301:errorcluster)  [unwired: 1 in, 1 out]
        n126 = Greater Than 0?(x=w277) -> (x > 0?=→"CW 2":bool)
        n127 = node-c288() -> ()  [unwired: 1 in, 1 out]
      }
      n128 = node-c288(w265) -> ()  [unwired: 1 out]
    }
    frame #3 {
      # "Close"
      n129 = call <vilib>:"Reset myRIO.vi"("error in (no error)"=w399) -> ("error out"=w385:errorcluster)  [unwired: 10 in]
      n130 = Concatenate Strings("OFF" ("데이터 입력"), "\r") -> (w393:string)
      n131 = Concatenate Strings("MV" ("데이터 입력"), "\r") -> (w392:string)
      n132 = Concatenate Strings(w393, w392, "V=0" ("데이터 입력"), "\r") -> (w389:string)
      n133 = TCP Write(connection ID=w388, data in=w389, error in (no error)=w387) -> (connection ID out=w398:refnum<k5>, error out=w386:errorcluster)  [unwired: 1 in, 1 out]
      n134 = TCP Close Connection(connection ID=w398, error in (no error)=w386) -> (error out=w383:errorcluster)  [unwired: 1 in, 1 out]
      n135 = Merge Errors(w385, w383) -> (→"error out 2":errorcluster)
    }
  }
  n136 = call "RC_receiver.vi"("Scale"="Speed scale", "baud rate (9600)"=u32 115200) -> ()  [unwired: 2 in]
  n137 = vi-ref "Control_type_change.vi"() -> ("vi reference"=w30:refnum<vi>)
  n138 = xnode "myRIO Register DI IRQ.xnode"("Channel Name"=tag "Button0 (Interrupt)", "Callback VI Reference"=w30, "Edge Count"=u32 1, "IRQ Number"=u8 0, "Digital Interrupt Type"=DI_IRQ_Type."Digital falling edge") -> ()  [unwired: 2 in, 1 out]
  n139 = node-c288() -> (w33:T3)  [unwired: 4 in]
  n140 = timed-loop {
    timing: w33 -> [_]
    timing-out: [_] -> w32
    stop <- w415 stop-if-true
    n141 = node-c288() -> ()  [unwired: 1 in, 1 out]
    n142 = global read "global.vi" "motion_command"() -> (w400:bool)
    n143 = xnode "Digital input (1 sample)"() -> ("control_state (A/DIO0 (Pin 11))"=w411:bool)  [unwired: 1 in, 1 out]
    n144 = global read "global.vi" "CTL_mode"() -> (w403:u8)
    n145 = global read "global.vi" "Speed/Torque"() -> (w412:bool)
    "S/T Control" <- w412
    n146 = global read "global.vi" "RC Control"() -> (w413:bool)
    "RC Control" <- w413
    n147 = global write "State2016.vi" "gear"(w403) -> ()
    n148 = global write "global.vi" "RC received"(w411) -> ()
    n149 = case shown="1, 2" w403 {
      tunnel: [w419 w421 w425 w429] -> w401
      tunnel: [w419 w420 w424 w428] -> w402
      frame 0, Default {
        n150 = Select(t="Torque", s="T/S", f="Speed") -> (s? t:f=w419:dbl)
        n151 = global write "global.vi" "Speed/Torque"("T/S") -> ()
      }
      frame 1, 2 {
        n152 = global read "motion_command.vi" "Angle Difference"() -> (w422:dbl)
        n153 = global read "motion_command.vi" "Goal speed"() -> (w423:dbl)
        n154 = formula code="float v_d = tan(delta)*v/4/0.33;\nL = v - v_d;\nR = v + v_d;"("v"=w423, "delta"=w422) -> ("R"=w420:dbl, "L"=w421:dbl)
      }
      frame 3 {
        n155 = global read "global.vi" "rc_ch2"() -> (w424:dbl)
        n156 = global read "global.vi" "rc_ch1"() -> (w425:dbl)
      }
      frame 4 {
        w426 = 500.0 ("y")
        n157 = global read "global.vi" "rc_ch1"() -> (w430:dbl)
        n158 = global read "global.vi" "rc_ch2"() -> (w427:dbl)
        n159 = Multiply(x=w426, y=w427) -> (x*y=w428:dbl)
        n160 = Multiply(x=w430, y=w426) -> (x*y=w429:dbl)
      }
    }
    n161 = xnode "LED"("LED1"=w412, "LED2"=w413, "LED3"=w400) -> ()  [unwired: 1 in, 1 out]
    n162 = global write "global.vi" "Stop"("Stop") -> ()
    n163 = xnode "Accelerometer"() -> ("X-Axis"=w409:dbl, "Y-Axis"=w410:dbl)  [unwired: 1 in, 1 out]
    n164 = global read "global.vi" "Stop"() -> (w415:bool)
    n165 = global write "State2016.vi" "lon_acc"(w409) -> ()
    n166 = global write "State2016.vi" "lat_acc"(w410) -> ()
    n167 = global read "State2016.vi" "front_right_wheel"() -> (w408:dbl)
    n168 = global read "State2016.vi" "front_left_wheel"() -> (w407:dbl)
    n169 = global write "global.vi" "Torque_L"(w401) -> ()
    n170 = global write "global.vi" "Speed_L"(w401) -> ()
    n171 = global write "global.vi" "Torque_R"(w402) -> ()
    n172 = global write "global.vi" "Speed_R"(w402) -> ()
    n173 = Add(x=w407, y=w408) -> (x+y=w406:dbl)
    n174 = Divide(x=w406, y=2.0) -> (x/y=w405:dbl)
    n175 = global write "State2016.vi" "velocity"(w405) -> ()
    n176 = node-c288() -> ()  [unwired: 1 in, 1 out]
  }
  n177 = node-c288(w16) -> ()  [unwired: 1 out]
  n178 = UDP Close(connection ID=w14, 8:w10) -> (error out=w9:errorcluster)  [unwired: 1 out]
  n179 = call <vilib>:"General Error Handler.vi"("error in (no error)"=w9) -> ()  [unwired: 10 in, 5 out]
  n180 = node-c288() -> (w8:T3)  [unwired: 4 in]
  n181 = UDP Open(9:-1 ("타임아웃 ms (25000)"), 11:u16 39001 ("포트")) -> (port=w4:refnum<k16>)  [unwired: 3 in, 2 out]
  n182 = timed-loop "state2016" {
    timing: w8 -> [_]
    timing-out: [_] -> w7
    tunnel: w4 -> [w600]
    tunnel: [w599] -> w3
    stop <- w544 stop-if-true
    w547 = 0.0  # lookahead_dist
    n183 = node-c288() -> ()  [unwired: 1 in, 1 out]
    n184 = global read "State2016.vi" "wheel_angle"() -> (w559:dbl)
    n185 = global read "State2016.vi" "velocity"() -> (w558:dbl)
    n186 = global read "State2016.vi" "front_left_wheel"() -> (w557:dbl)
    n187 = global read "State2016.vi" "front_right_wheel"() -> (w556:dbl)
    n188 = global read "State2016.vi" "rear_left_wheel"() -> (w555:dbl)
    n189 = global read "State2016.vi" "rear_right_wheel"() -> (w554:dbl)
    n190 = global read "State2016.vi" "yaw_rate"() -> (w553:dbl)
    n191 = global read "State2016.vi" "lon_acc"() -> (w552:dbl)
    n192 = global read "State2016.vi" "lat_acc"() -> (w551:dbl)
    n193 = global read "State2016.vi" "gear"() -> (w550:dbl)
    n194 = global read "State2016.vi" "emergency"() -> (w545:bool)
    n195 = Boolean To (0,1)(Boolean=w545) -> (0, 1=w546:i16)
    n196 = Number To Fractional String(number=w559) -> (F-format string=w592:string)  [unwired: 3 in]
    n197 = Number To Fractional String(number=w558) -> (F-format string=w591:string)  [unwired: 3 in]
    n198 = Number To Fractional String(number=w557) -> (F-format string=w575:string)  [unwired: 3 in]
    n199 = Number To Fractional String(number=w556) -> (F-format string=w573:string)  [unwired: 3 in]
    n200 = Number To Fractional String(number=w555) -> (F-format string=w571:string)  [unwired: 3 in]
    n201 = Number To Fractional String(number=w554) -> (F-format string=w569:string)  [unwired: 3 in]
    n202 = Number To Fractional String(number=w553) -> (F-format string=w589:string)  [unwired: 3 in]
    n203 = Number To Fractional String(number=w552) -> (F-format string=w587:string)  [unwired: 3 in]
    n204 = Number To Fractional String(number=w551) -> (F-format string=w584:string)  [unwired: 3 in]
    n205 = Number To Fractional String(number=w550) -> (F-format string=w580:string)  [unwired: 3 in]
    n206 = Number To Fractional String(number=w547) -> (F-format string=w577:string)  [unwired: 3 in]
    n207 = Number To Fractional String(number=w546) -> (F-format string=w565:string)  [unwired: 3 in]
    n208 = call <vilib>:"Space Constant.vi"() -> ("String"=w594:string)
    n209 = call <vilib>:"Space Constant.vi"() -> ("String"=w593:string)
    n210 = call <vilib>:"Space Constant.vi"() -> ("String"=w576:string)
    n211 = call <vilib>:"Space Constant.vi"() -> ("String"=w574:string)
    n212 = call <vilib>:"Space Constant.vi"() -> ("String"=w572:string)
    n213 = call <vilib>:"Space Constant.vi"() -> ("String"=w570:string)
    n214 = call <vilib>:"Space Constant.vi"() -> ("String"=w590:string)
    n215 = call <vilib>:"Space Constant.vi"() -> ("String"=w588:string)
    n216 = call <vilib>:"Space Constant.vi"() -> ("String"=w585:string)
    n217 = call <vilib>:"Space Constant.vi"() -> ("String"=w581:string)
    n218 = call <vilib>:"Space Constant.vi"() -> ("String"=w578:string)
    n219 = call <vilib>:"Space Constant.vi"() -> ("String"=w564:string)
    n220 = Concatenate Strings(w592, w594) -> (w563:string)
    n221 = Concatenate Strings(w591, w593) -> (w562:string)
    n222 = Concatenate Strings(w575, w576) -> (w561:string)
    n223 = Concatenate Strings(w573, w574) -> (w560:string)
    n224 = Concatenate Strings(w571, w572) -> (w568:string)
    n225 = Concatenate Strings(w569, w570) -> (w567:string)
    n226 = Concatenate Strings(w589, w590) -> (w586:string)
    n227 = Concatenate Strings(w587, w588) -> (w582:string)
    n228 = Concatenate Strings(w584, w585) -> (w583:string)
    n229 = Concatenate Strings(w580, w581) -> (w579:string)
    n230 = Concatenate Strings(w577, w578) -> (w548:string)
    n231 = Concatenate Strings(w565, w564) -> (w549:string)
    n232 = String To IP(1:"192.168.3.70" ("이름")) -> (0:w597:u32)
    n233 = global read "global.vi" "Stop"() -> (w544:bool)
    n234 = Concatenate Strings(w563, w562, w561, w560, w568, w567, w586, w582, w583, w579, w548, w549, "\r") -> (w595:string)
    n235 = node-c288() -> ()  [unwired: 1 in, 1 out]
    n236 = UDP Write(address=w597, port or service name=u16 39001 ("포트 또는 서비스 이름"), connection ID=w600, data in=w595, 9:1000 ("타임아웃 ms (25000)")) -> (3:w599:refnum<k16>)  [unwired: 1 in, 1 out]
  }
  n237 = node-c288(w32) -> ()  [unwired: 1 out]
  n238 = node-c288(w7) -> ()  [unwired: 1 out]
  n239 = UDP Close(connection ID=w3) -> ()  [unwired: 1 in, 2 out]
